vi "PH_TKTDS-30xx.Configure Trigger.vi"(0 "i ref in":refnum<vi>, 2 "Trigger Configuration":T1={"Source"="CH1", "Slope"=0, "Level [V]"=0.0} {"Level [V]" format="%#_6p"}, 5 "error IO":errorcluster) -> (14 "i ref out":refnum<vi>, 19 "error out":errorcluster)   [LabVIEW 2014, in "PH_TKTDS-30xx.lvlib"]
doc: "If the connection is established, the trigger configuration is set and written to own attributes as well as the errors."
uses:
  PH_TKTDS-30xx.lvlib
  PH_TKTDS-30xx.Trigger Config.ctl
  non_GPL/instr.lib/tktds3032-PHELIX/tktds3032-PHELIX - Driver np.lvlib
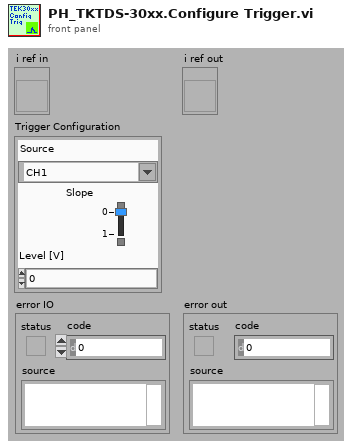
[diagram p1: front panel]
types:
  T1 = typedef "PH_TKTDS-30xx.lvlib/PH_TKTDS-30xx.Trigger Config.ctl" = cluster{"Source":string, "Slope":i32, "Level [V]":dbl}
  T2 = typedef "PH_TKTDS-30xx.lvlib/PH_TKTDS-30xx.i attribute.ctl" = cluster{"Default VISA Resource":string, "VISA Resource Name":refnum<visa-resource-name>, "Revision":cluster{"Instrument Driver":string, "Instrument Firmware":string}, "Selftest":cluster{"Result":u32, "Message":string}, "Channels":T3[], "Trigger Configuration":T1, "Acquisition Configuration":T4, "Fetched Waveforms":T5[], "GUI Refs":T6, "GUI Refs Channels":refnum<vi>[], "State":T7, "Error Message":string, "Allow Prdc Loop?":bool}
  T3 = typedef "PH_TKTDS-30xx.lvlib/PH_TKTDS-30xx.Channel Config.ctl" = cluster{"Channel Name":string, "Input Impedance":string, "Max Input Frequency":string, "Vertical Coupling":i32, "Channel Enabled":bool, "Probe Attenuation":dbl, "Vertical Range":dbl, "Vertical Offset":dbl}
  T4 = typedef "PH_TKTDS-30xx.lvlib/PH_TKTDS-30xx.Acquisition Config.ctl" = cluster{"Time base":dbl, "Record Length":u16, "Start Time":dbl, "Type":i32, "Continuous":bool}
  T5 = typedef "PH_TKTDS-30xx.lvlib/PH_TKTDS-30xx.fetched Waveform.ctl" = cluster{"Source":string, "Actual Points":u32, "Initial X":dbl, "X Increment":dbl, "Waveform Array":dbl[]}
  T6 = typedef "PH_TKTDS-30xx.lvlib/PH_TKTDS-30xx.GUI Refs.ctl" = cluster{"Trigger":refnum<vi>, "Acquisition":refnum<vi>, "Graph":refnum<vi>, "State":refnum<vi>, "Delete":refnum<vi>, "Channel to be positioned":refnum<vi>, "Postion":refnum<vi>, "Display Intensity":refnum<vi>, "VISA Resource":refnum<vi>}
  T7 = typedef "PH_StatusHandler.lvlib/PH_StatusHandler.Status.ctl" = i16
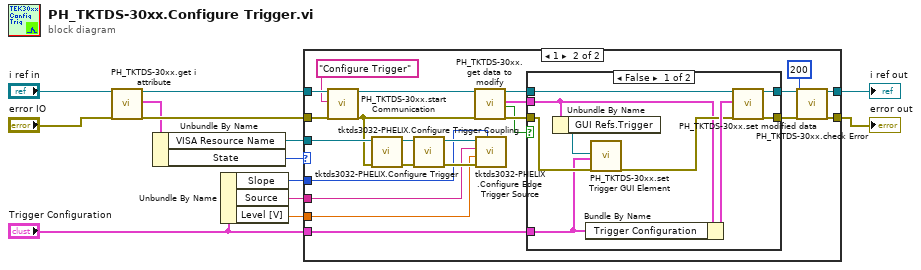
[diagram p0: block diagram]
diagram:
  n1 = call "PH_TKTDS-30xx.get i attribute.vi"("i ref in"="i ref in", "error in (no error)"="error IO") -> ("i ref out"=w8:refnum<vi>, "i attribute"=w10:T2, "error out"=w12:errorcluster)  [unwired: 15 in]
  n2 = Unbundle By Name(w10) -> ("VISA Resource Name"=w11:refnum<visa-resource-name>, "State"=w3:T7)
  n3 = Unbundle By Name("Trigger Configuration") -> ("Slope"=w1:i32, "Source"=w5:string, "Level [V]"=w4:dbl)
  n4 = case shown="1" w3 {
    tunnel: w8 -> [w15 w23]
    tunnel: w11 -> [_ w31]
    tunnel: [w14 w21] -> w6
    tunnel: w12 -> [w14 w25]
    tunnel: [w15 w19] -> w13
    tunnel: w5 -> [_ w28]
    tunnel: w1 -> [_ w26]
    tunnel: w4 -> [_ w27]
    tunnel: "Trigger Configuration" -> [_ w16]
    frame Default {
    }
    frame 1 {
      n5 = call "PH_TKTDS-30xx.start Communication.vi"("i ref in"=w23, "Action"="Configure Trigger", "error in"=w25) -> ("i ref out"=w22:refnum<vi>, "error out"=w24:errorcluster)  [unwired: 15 in]
      n6 = call "tktds3032-PHELIX.Configure Trigger.vi"("error in (no error)"=w24, "VISA Resource Name"=w31) -> ("error out"=w30:errorcluster, "VISA Resource Name Out"=w32:refnum<visa-resource-name>)  [unwired: 8 in]
      n7 = call "tktds3032-PHELIX.Configure Trigger Coupling.vi"("error in (no error)"=w30, "VISA Resource Name"=w32) -> ("error out"=w29:errorcluster, "VISA Resource Name Out"=w33:refnum<visa-resource-name>)  [unwired: 8 in]
      n8 = call "PH_TKTDS-30xx.get data to modify.vi"("i ref in"=w22, "error in (no error)"=w24) -> ("i ref out"=w36:refnum<vi>, "i attribute"=w34:T2, "timed out"=w35:bool, "error out"=w37:errorcluster)  [unwired: 14 in]
      n9 = call "tktds3032-PHELIX.Configure Edge Trigger Source.vi"("Trigger Slope (Positive)"=w26, "error in (no error)"=w29, "Trigger Level (0.0 V)"=w27, "Trigger Source (Channel 1)"=w28, "VISA Resource Name"=w33) -> ()  [unwired: 5 in, 2 out]
      n10 = case shown="False" w35 {
        tunnel: [w47 w48] -> w38
        tunnel: w37 -> [w46 w48]
        tunnel: w36 -> [w45 w49]
        tunnel: [w44 w49] -> w20
        tunnel: w34 -> [w41 _]
        tunnel: w16 -> [w39 _]
        frame False {
          n11 = Unbundle By Name(w41) -> ("GUI Refs.Trigger"=w40:refnum<vi>)
          n12 = Bundle By Name(cluster=w41, "Trigger Configuration"=w39) -> (w43:T2)
          n13 = call "PH_TKTDS-30xx.set Trigger GUI Element.vi"("Ref Trigger Config"=w40, "Trigger Config"=w39, "error in"=w46) -> ("error out"=w42:errorcluster)  [unwired: 16 in]
          n14 = call "PH_TKTDS-30xx.set modified data.vi"("i ref in"=w45, "i attribute"=w43, "error in (no error)"=w42) -> ("i ref out"=w44:refnum<vi>, "error out"=w47:errorcluster)  [unwired: 15 in]
        }
        frame True {
        }
      }
      n15 = call "PH_TKTDS-30xx.check Error.vi"("i ref in"=w20, "Waiting Time [ms]"=u32 200, "error in"=w38) -> ("i ref out"=w19:refnum<vi>, "error out"=w21:errorcluster)  [unwired: 15 in]
    }
  }
  "i ref out" <- w13
  "error out" <- w6
